vi "TxBfrPkt - Add Packet.vi"(5 "Add Port Channel?":bool, 7 "Ext Buffer?":bool, 8 "error in (no error)":errorcluster, 9 "New Packet ID":i32, 10 "New Packet Name":string, 11 "Item Ref in":T1=18446744073709551615 format="%.0x") -> (0 "error out":errorcluster, 2 "New Packet Ref":T1=18446744073709551615 format="%.0x", 3 "Item Ref Out":T1=18446744073709551615 format="%.0x")   [LabVIEW 2016, in "UDP-Custom-Device System Explorer.lvlib"]
uses:
  UDP-Custom-Device System Explorer.lvlib
  <vilib>/NI Veristand/Custom Device API/Custom Device Item Ref.ctl
  Shared/Constants.vi
  Shared/UDP-Custom-Device Shared.lvlib
  Property Accessors/Shared Section Accessors.lvlib
  <vilib>/NI VeriStand/Custom Device API/Custom Device API.lvlib
  Property Accessors/Shared Packet Accessors.lvlib
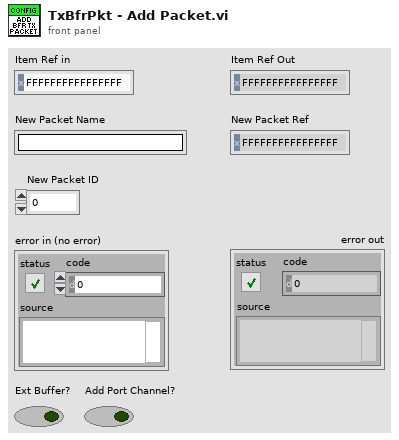
[diagram p1: front panel]
types:
  T1 = typedef "Custom Device API.lvlib/Custom Device Item Ref.ctl" = u64
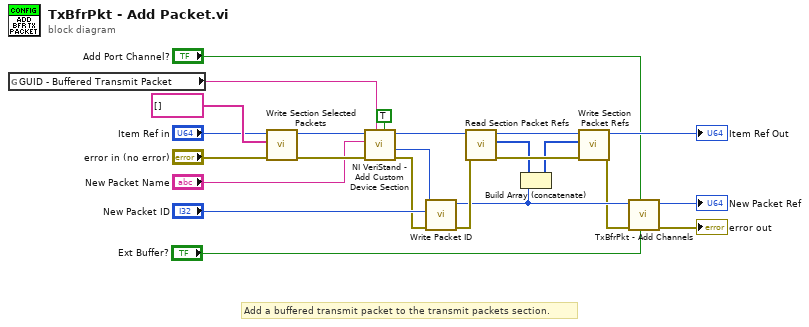
[diagram p0: block diagram]
diagram:
  # "Add a buffered transmit packet to the transmit packets section."
  n1 = global read "Constants.vi" "GUID - Buffered Transmit Packet"() -> (w18:string)
  n2 = call "Write Section Selected Packets.vi"("error in (no error)"="error in (no error)", "Selected Packets"=string[] [] ("Value"), "Node Ptr"="Item Ref in") -> ("error out"=w19:errorcluster, "Node Ptr out"=w20:T1)  [unwired: 7 in]
  n3 = call <vilib>:"NI VeriStand - Add Custom Device Section.vi"("Highlight? (F)"=TRUE, "GUID (Default Section)"=w18, "error in (no error)"=w19, "Section Name"="New Packet Name", "Parent Ref in"=w20) -> ("error out"=w8:errorcluster, "Section Ptr"=w10:T1, "Parent Ref out"=w11:T1)  [unwired: 3 in, 1 out]
  n4 = call "Write Packet ID.vi"("error in (no error)"=w8, "Packet ID"="New Packet ID", "Node Ptr"=w10) -> ("error out"=w16:errorcluster, "Node Ptr out"=w6:T1)  [unwired: 7 in]
  n5 = call "Read Section Packet Refs.vi"("error in (no error)"=w16, "Node Ptr"=w11) -> ("error out"=w15:errorcluster, "Dependent Node Refs"=w13:T1[], "Node Ptr out"=w12:T1)  [unwired: 7 in]
  n6 = Build Array (concatenate)(w13, w6) -> (w14:T1[])
  n7 = call "Write Section Packet Refs.vi"("error in (no error)"=w15, "Dependent Node Refs"=w14, "Node Ptr"=w12) -> ("error out"=w5:errorcluster, "Node Ptr out"=→"Item Ref Out":T1)  [unwired: 7 in]
  n8 = call "TxBfrPkt - Add Channels.vi"("Ext Buffer?"="Ext Buffer?", "Add Port Channel?"="Add Port Channel?", "error in (no error)"=w5, "Node Ptr"=w6) -> ("error out"=→"error out":errorcluster, "Node Ptr out"=→"New Packet Ref":T1)  [unwired: 6 in]
